vi "Add_Int.vi"(9 "Value":i32, 10 "Key":string, 11 "Keyword Array":T1[](array[typedef])) -> (3 "Keyword Array Out":T1[](array[typedef]))   [LabVIEW 2013, in "Advanced Plotting Toolkit.lvlib"]
uses:
  Advanced Plotting Toolkit.lvlib
  KeyValue.ctl
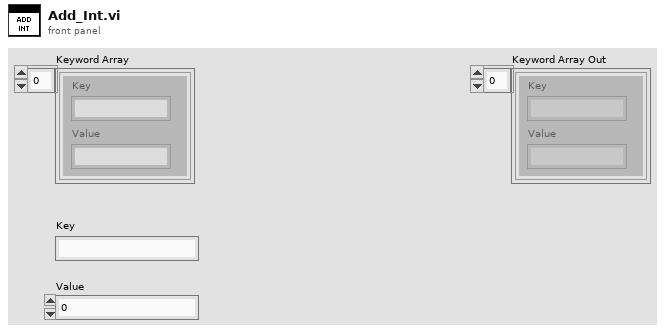
[diagram p1: front panel]
types:
  T1 = typedef "Advanced Plotting Toolkit.lvlib/KeyValue.ctl" = cluster{"Key":string, "Value":string}
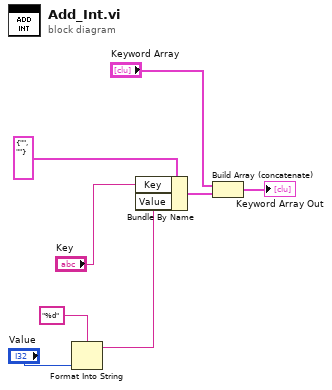
[diagram p0: block diagram]
diagram:
  n1 = Format Into String(format string="%d", "Value") -> (resulting string=w1:string)  [unwired: 2 in, 1 out]
  n2 = Bundle By Name(cluster=T1 {"Key"="", "Value"=""} ("KeyValue"), "Key"="Key", "Value"=w1) -> (w6:T1)
  n3 = Build Array (concatenate)("Keyword Array", w6) -> (→"Keyword Array Out":T1[])
